vi "createModbusRxDataFIFO.vi"(8 "error in (no error)":errorcluster, 11 "Boot in":refnum<class "Boot.lvclass">) -> (0 "error out":errorcluster, 2 "ReadU16FIFO":refnum<class "IReadU16FIFO.lvclass">, 3 "Boot out":refnum<class "Boot.lvclass">)   [LabVIEW 2016, in "Boot.lvclass"]
uses:
  Boot.lvclass
  Common_RT_FPGA/IReadU16FIFO/IReadU16FIFO.lvclass
  Resources/ModbusRxDataFIFO/ModbusRxDataFIFO.lvclass
  D:/Code/ts_M1M3Support/Common_RT_FPGA/IReadU16FIFO/IReadU16FIFO.lvclass
  Boot.lvclass/Boot.ctl
  Resources/ModbusRxDataFIFO/ModbusRxDataFIFO.lvclass/ModbusRxDataFIFO.ctl
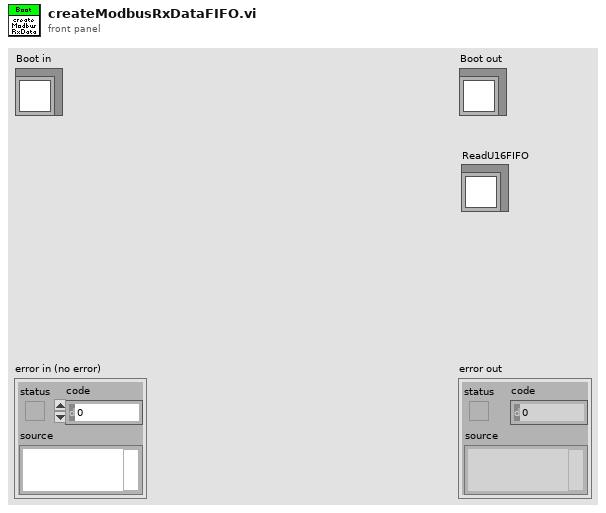
[diagram p1: front panel]
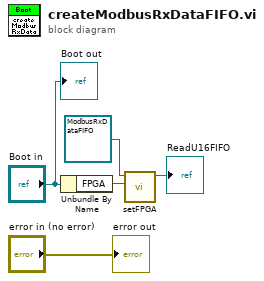
[diagram p0: block diagram]
diagram:
  n1 = Unbundle By Name("Boot in") -> ("FPGA"=w2:refnum<class "FPGA.lvclass">)
  n2 = call "setFPGA.vi"("FPGA"=w2, "ModbusRxDataFIFO in"=refnum<class "ModbusRxDataFIFO.lvclass"> refnum ("ModbusRxDataFIFO.lvclass")) -> ("ModbusRxDataFIFO out"=→"ReadU16FIFO":refnum<class "ModbusRxDataFIFO.lvclass">)  [unwired: 9 in]
  "error out" <- "error in (no error)"
  "Boot out" <- "Boot in"
